vi "target_main.vi"() -> ()   [LabVIEW 2023]
uses:
  <vilib>/Platform/TimedLoop/XDataNode/timing_clust.ctl
  <vilib>/Platform/TimedLoop/XDataNode/nitl_modes.ctl
  <vilib>/Platform/TimedLoop/XDataNode/wakeup.ctl
  <vilib>/rvi/Emulation/niFpgaGetClockAttributes.vi
  <vilib>/rvi/Emulation/niFpgaSctlEmulationGetInTimedLoop.vi
  <vilib>/rvi/Emulation/niFpgaEmulationReportErrorSimple.vi
  <vilib>/rvi/Emulation/niFpgaProcessEmulError.vi
  <vilib>/eio/utilities/niEioResolveVilibRelativePath.vi
  <vilib>/rvi/interface/RandomDataEmulation/niFpgaRandomDataHandleErrors.vi
  <vilib>/rvi/Emulation/niFpgaCriticalErrorInLSC.vi
  <vilib>/rvi/eio/common/nirviEmuTemplateMethod_errors.vi
  <vilib>/rvi/DataTransferAndStorage/Container/XNode/niFpgaContainer.xnode
  <vilib>/rvi/interface/RandomDataEmulation/nirviRandomDataFpgaReadWriteTemplate.vi
  <vilib>/Platform/TimedLoop/XDataNode/XDataNode.xnode
  <vilib>/eio/EIONode/EIONode.xnode
  <vilib>/Platform/TimedLoop/XDataNode/XDNodeRunTimeDep.lvlib
panel:
  out "pin 6":sgl
  out "pin 5":sgl
  out "pin 4":sgl
  out "pin 2":sgl
  out "pin 3":sgl
  out "pin 1":sgl format="%.2f"
  in  "FPGA FIFO Status Update (ms)":u32=100 caption="FPGA FIFO Status Update (mSec)"
  in  "Action Abort":bool
  in  "Status Code":u8
  in  "Analogue 2":u32
  in  "Analogue 1":u32
  in  "Analogue 0":u32
  in  "Digital 0":u32
  in  "Analogue 2 Read":bool
  in  "Analogue 1 Read":bool
  in  "Analogue 0 Read":bool
  in  "Digital 0 Read":bool
  in  "Action: Analogue 2":u64
  in  "Action: Analogue 1":u64
  in  "Action: Analogue 0":u64
  in  "Action: Digital 0":u64
  in  "FPGA Tick Reset":bool
  in  "FPGA Status Update Loop Time (ms)":u32=100 caption="FPGA Execution Status Update (mSec)"
  out "FPGA Target Clock Tick":u32
  # "Current Actions"
  # "Action Execution"
  # "FIFO Read Request"
  # "UDP: FPGA Line Status"
  # "Analogue 0: Optical Switch Pin Status"
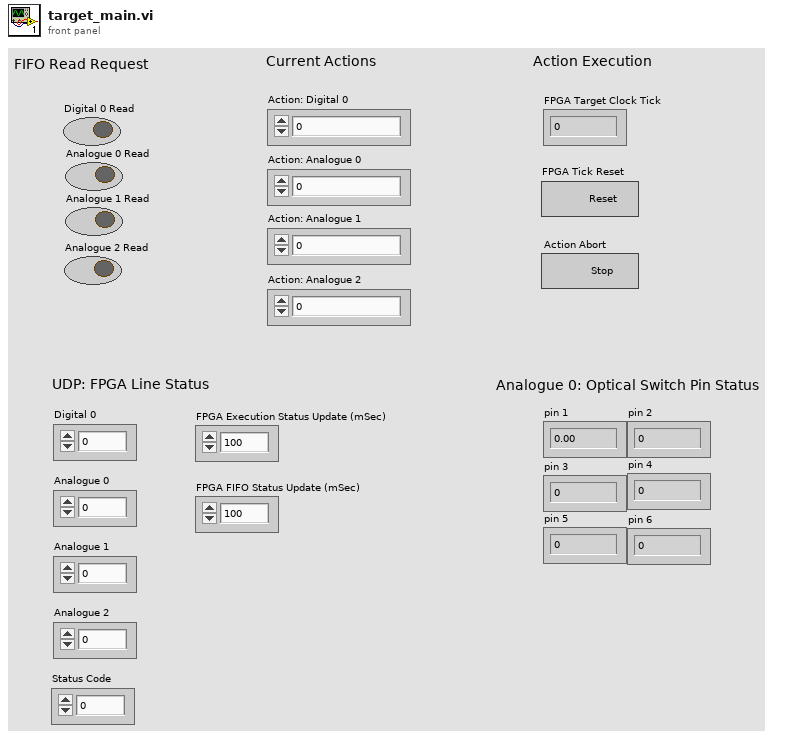
[diagram p1: front panel]
types:
  T1 = typedef "XDNodeRunTimeDep.lvlib/timing_clust.ctl" = cluster{"Expected End [f-1]":u64, "Actual End [f-1]":u64, "Finished Late? [f-1]":bool, "Expected End [i-1]":u64, "Actual End [i-1]":u64, "Finished Late? [i-1]":bool, "Expected Start [i]":u64, "Actual Start [i]":u64, "Expected Start [f]":u64, "Actual Start [f]":u64, "Source Name":string, "Structure Name":string, "Period":i64, "Deadline":i64, "Offset":i64, "Start":i64, "Priority":i32, "Timeout":i32, "Mode":T2, "Wakeup Reason":T3, "Error":errorcluster, "Source Type":string, "Secondary Source Type":string, "Global End Time":u64, "Global Start Time":u64, "Frame Duration":u64, "Iteration Duration":u64, "Assigned CPU":i32, "I/O Scan Engine Mode":u32}
  T2 = typedef "XDNodeRunTimeDep.lvlib/nitl_modes.ctl" = enum32{"No Change", "Process missed periods, maintain original phase", "Discard missed periods, maintain original phase", "Process missed periods, ignore original phase", "Discard missed periods, ignore original phase"}
  T3 = typedef "XDNodeRunTimeDep.lvlib/wakeup.ctl" = enum32{"Normal", "Aborted", "Asynchronous wakeup", "Timing source error", "Timed loop error", "Timeout"}
  T4 = cluster{"pin 1":sgl, "pin 3":sgl, "pin 5":sgl, "pin 6":sgl, "pin 2":sgl, "pin 4":sgl}[]
  T5 = cluster{"pin 1":sgl, "pin 3":sgl, "pin 5":sgl, "pin 6":sgl, "pin 2":sgl, "pin 4":sgl}
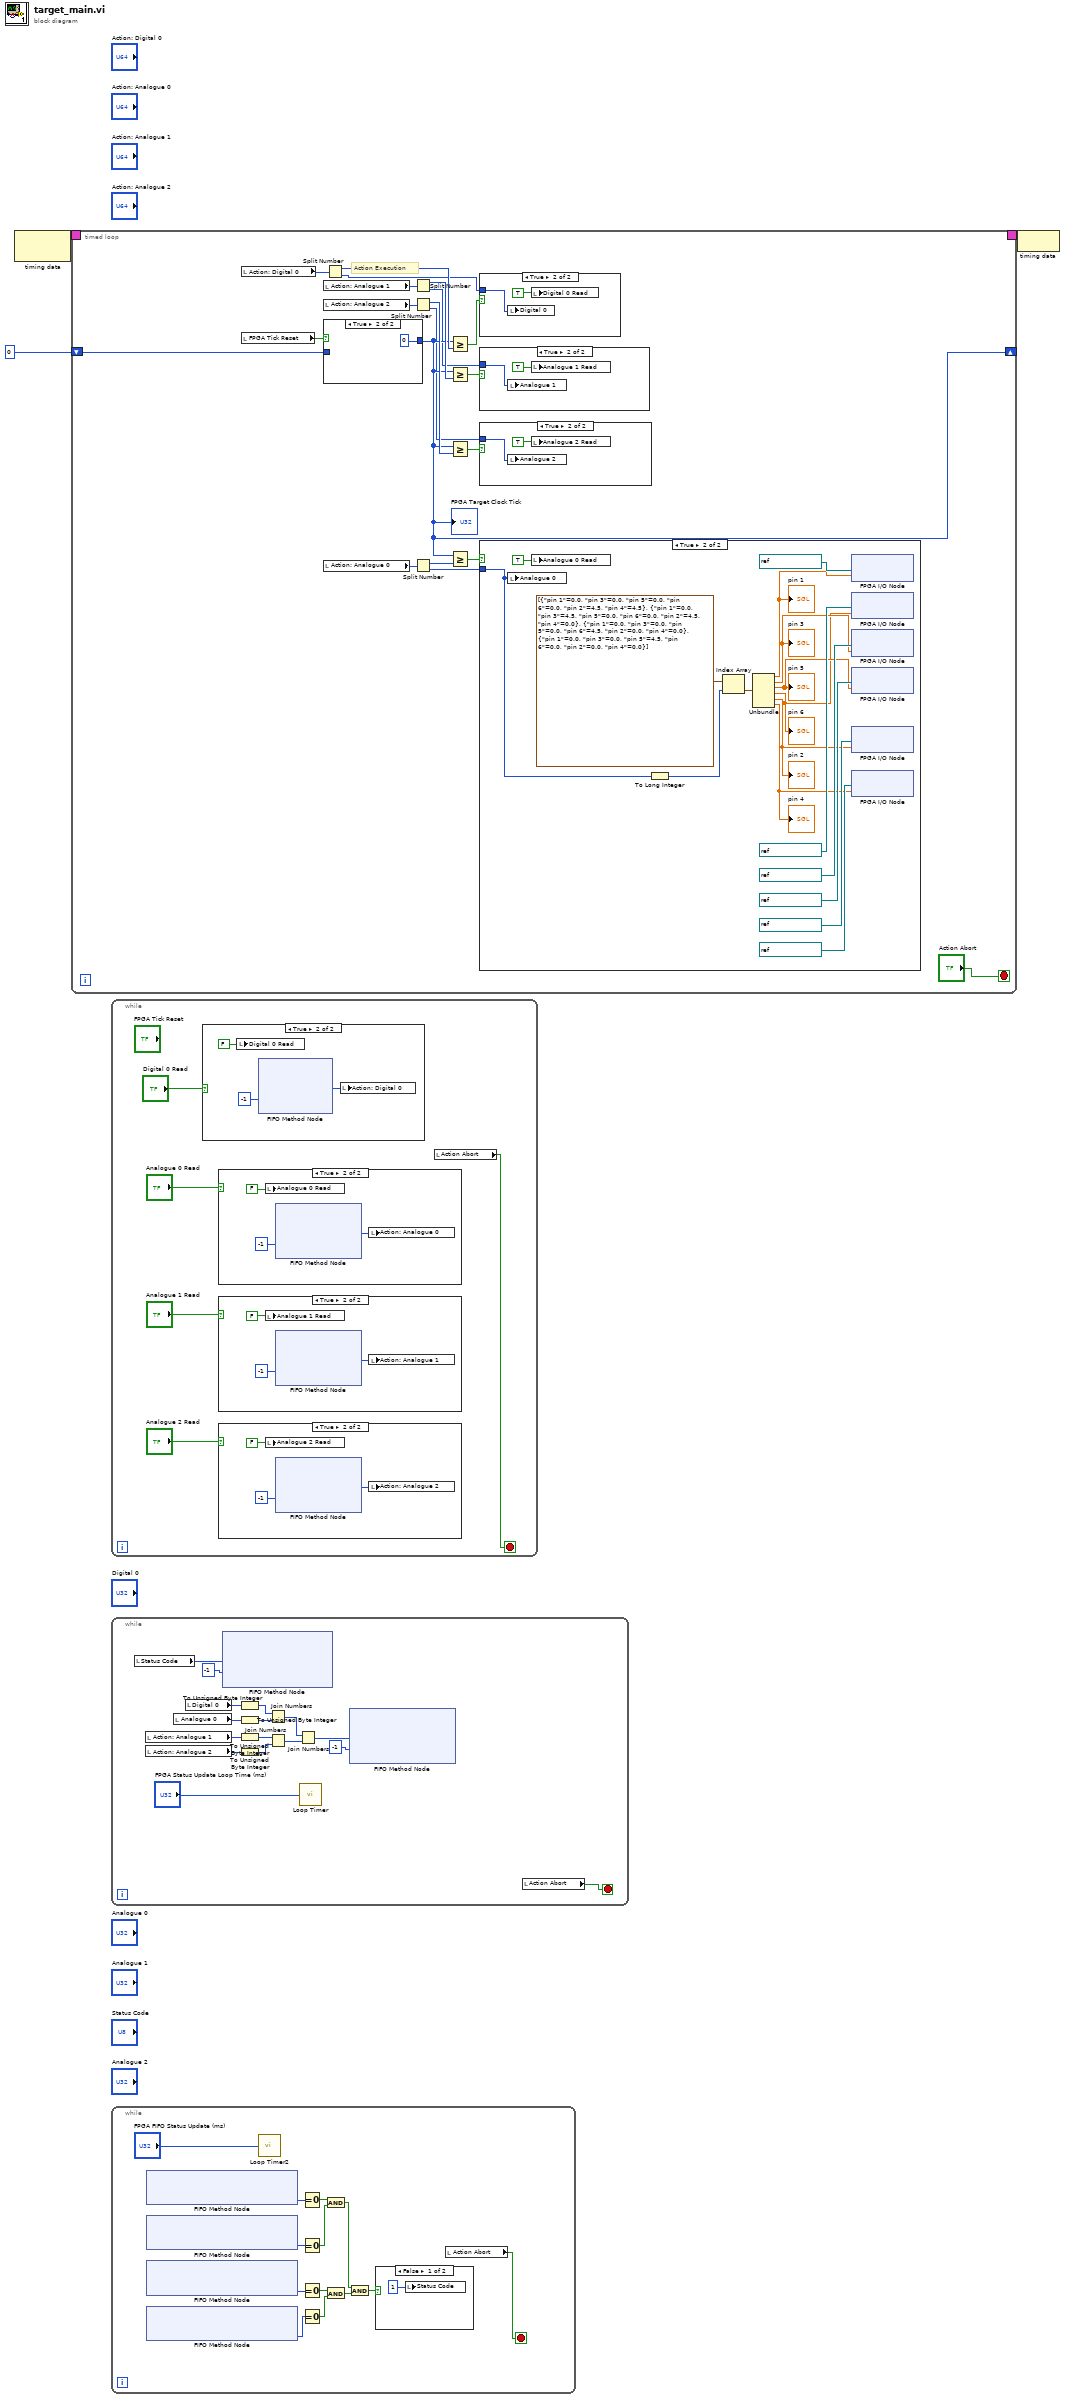
[diagram p0: block diagram]
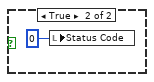
[diagram p2: hidden frame]
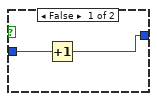
[diagram p7: hidden frame]
diagram:
  n1 = node-c288() -> (w3:T1)  [unwired: 1 in]
  n2 = timed-loop {
    timing: w3 -> [_]
    timing-out: [_] -> w2
    shift-right: [w13] -> _
    shift-left: u32 0 -> [w22]
    stop <- "Action Abort" stop-if-true
    # "Action Execution"
    n3 = local read "Action: Digital 0"() -> (w21:u64)
    n4 = local read "FPGA Tick Reset"() -> (w23:bool)
    n5 = local read "Action: Analogue 1"() -> (w19:u64)
    n6 = local read "Action: Analogue 2"() -> (w18:u64)
    n7 = case shown="True" w23 {
      tunnel: [w48 u32 0] -> w13
      tunnel: w22 -> [w47 _]
      frame False {
        n8 = Increment(x=w47) -> (x+1=w48:u32)
      }
      frame True {
      }
    }
    "FPGA Target Clock Tick" <- w13
    n9 = local read "Action: Analogue 0"() -> (w20:u64)
    n10 = Split Number(x=w21) -> (hi(x)=w17:u32, lo(x)=w11:u32)
    n11 = Split Number(x=w19) -> (hi(x)=w15:u32, lo(x)=w7:u32)
    n12 = Split Number(x=w18) -> (hi(x)=w14:u32, lo(x)=w5:u32)
    n13 = Split Number(x=w20) -> (hi(x)=w16:u32, lo(x)=w9:u32)
    n14 = Greater Or Equal?(x=w13, y=w17) -> (x >= y?=w12:bool)
    n15 = Greater Or Equal?(x=w13, y=w15) -> (x >= y?=w8:bool)
    n16 = Greater Or Equal?(x=w13, y=w14) -> (x >= y?=w6:bool)
    n17 = Greater Or Equal?(x=w13, y=w16) -> (x >= y?=w10:bool)
    n18 = case shown="True" w12 {
      tunnel: w11 -> [_ w46]
      frame False {
      }
      frame True {
        n19 = local write "Digital 0"(w46) -> ()
        n20 = local write "Digital 0 Read"(TRUE) -> ()
      }
    }
    n21 = case shown="True" w8 {
      tunnel: w7 -> [_ w27]
      frame False {
      }
      frame True {
        n22 = local write "Analogue 1"(w27) -> ()
        n23 = local write "Analogue 1 Read"(TRUE ("Analogue 1 Read")) -> ()
      }
    }
    n24 = case shown="True" w6 {
      tunnel: w5 -> [_ w25]
      frame False {
      }
      frame True {
        n25 = local write "Analogue 2"(w25) -> ()
        n26 = local write "Analogue 2 Read"(TRUE ("Analogue 2 Read")) -> ()
      }
    }
    n27 = case shown="True" w10 {
      tunnel: w9 -> [_ w28]
      frame False {
      }
      frame True {
        n28 = local write "Analogue 0"(w28) -> ()
        n29 = local write "Analogue 0 Read"(TRUE ("Analogue 0 Read")) -> ()
        n30 = To Long Integer(number=w28) -> (32bit integer=w29:i32)
        n31 = Index Array(array=T4 [{"pin 1"=0.0, "pin 3"=0.0, "pin 5"=0.0, "pin 6"=0.0, "pin 2"=4.5, "pin 4"=4.5}, {"pin 1"=0.0, "pin 3"=4.5, "pin 5"=0.0, "pin 6"=0.0, "pin 2"=4.5, "pin 4"=0.0}, {"pin 1"=0.0, "pin 3"=0.0, "pin 5"=0.0, "pin 6"=4.5, "pin 2"=0.0, "pin 4"=0.0}, {"pin 1"=0.0, "pin 3"=0.0, "pin 5"=4.5, "pin 6"=0.0, "pin 2"=0.0, "pin 4"=0.0}], index=w29) -> (element=w36:T5)
        n32 = Unbundle(w36) -> ("pin 1"=w35:sgl, "pin 3"=w34:sgl, "pin 5"=w31:sgl, "pin 6"=w30:sgl, "pin 2"=w33:sgl, "pin 4"=w32:sgl)
        "pin 1" <- w35
        "pin 3" <- w34
        "pin 2" <- w33
        "pin 4" <- w32
        "pin 5" <- w31
        "pin 6" <- w30
        n33 = xnode "FPGA I/O Node"("I/O Item"=w35, "FPGA I/O In"=refnum<k21> "Mod3/AO0") -> ()  [unwired: 1 out]
        n34 = xnode "FPGA I/O Node"("I/O Item"=w30, "FPGA I/O In"=refnum<k21> "Mod3/AO5") -> ()  [unwired: 1 out]
        n35 = xnode "FPGA I/O Node"("I/O Item"=w34, "FPGA I/O In"=refnum<k21> "Mod3/AO2") -> ()  [unwired: 1 out]
        n36 = xnode "FPGA I/O Node"("I/O Item"=w31, "FPGA I/O In"=refnum<k21> "Mod3/AO4") -> ()  [unwired: 1 out]
        n37 = xnode "FPGA I/O Node"("I/O Item"=w33, "FPGA I/O In"=refnum<k21> "Mod3/AO1") -> ()  [unwired: 1 out]
        n38 = xnode "FPGA I/O Node"("I/O Item"=w32, "FPGA I/O In"=refnum<k21> "Mod3/AO3") -> ()  [unwired: 1 out]
      }
    }
  }
  n39 = while {
    stop <- w52 stop-if-true
    n40 = case shown="True" "Digital 0 Read" {
      frame False {
      }
      frame True {
        n41 = local write "Digital 0 Read"(FALSE) -> ()
        n42 = xnode ("FIFO Method Node")("Timeout"=-1) -> ("Element"=w68:u64)  [unwired: 1 in, 2 out]
        n43 = local write "Action: Digital 0"(w68) -> ()
      }
    }
    n44 = case shown="True" "Analogue 0 Read" {
      frame False {
      }
      frame True {
        n45 = local write "Analogue 0 Read"(FALSE) -> ()
        n46 = xnode ("FIFO Method Node")("Timeout"=-1) -> ("Element"=w65:u64)  [unwired: 1 in, 2 out]
        n47 = local write "Action: Analogue 0"(w65) -> ()
      }
    }
    n48 = case shown="True" "Analogue 1 Read" {
      frame False {
      }
      frame True {
        n49 = local write "Analogue 1 Read"(FALSE) -> ()
        n50 = xnode ("FIFO Method Node")("Timeout"=-1) -> ("Element"=w62:u64)  [unwired: 1 in, 2 out]
        n51 = local write "Action: Analogue 1"(w62) -> ()
      }
    }
    n52 = case shown="True" "Analogue 2 Read" {
      frame False {
      }
      frame True {
        n53 = local write "Analogue 2 Read"(FALSE) -> ()
        n54 = xnode ("FIFO Method Node")("Timeout"=-1) -> ("Element"=w59:u64)  [unwired: 1 in, 2 out]
        n55 = local write "Action: Analogue 2"(w59) -> ()
      }
    }
    n56 = local read "Action Abort"() -> (w52:bool)
  }
  n57 = while {
    stop <- w81 stop-if-true
    n58 = local read "Status Code"() -> (w82:u8)
    n59 = local read "Action: Analogue 1"() -> (w78:u64)
    n60 = local read "Action: Analogue 2"() -> (w77:u64)
    n61 = local read "Analogue 0"() -> (w79:u32)
    n62 = local read "Digital 0"() -> (w80:u32)
    n63 = xnode ("FIFO Method Node")("Element"=w82, "Timeout"=-1) -> ()  [unwired: 1 in, 2 out]
    n64 = To Unsigned Byte Integer(number=w80) -> (unsigned 8bit integer=w76:u8)
    n65 = To Unsigned Byte Integer(number=w79) -> (unsigned 8bit integer=w75:u8)
    n66 = To Unsigned Byte Integer(number=w78) -> (unsigned 8bit integer=w74:u8)
    n67 = To Unsigned Byte Integer(number=w77) -> (unsigned 8bit integer=w73:u8)
    n68 = Join Numbers(hi=w76, lo=w75) -> ((hi.lo)=w71:u16)
    n69 = Join Numbers(hi=w74, lo=w73) -> ((hi.lo)=w72:u16)
    n70 = Join Numbers(hi=w71, lo=w72) -> ((hi.lo)=w70:u32)
    n71 = call "Loop Timer"("Count(mSec)"="FPGA Status Update Loop Time (ms)") -> ()  [unwired: 1 out]
    n72 = xnode ("FIFO Method Node")("Element"=w70, "Timeout"=-1) -> ()  [unwired: 1 in, 2 out]
    n73 = local read "Action Abort"() -> (w81:bool)
  }
  n74 = while {
    stop <- w97 stop-if-true
    n75 = xnode ("FIFO Method Node")() -> ("Number of Elements to Read"=w96:u32)  [unwired: 1 in, 1 out]
    n76 = xnode ("FIFO Method Node")() -> ("Number of Elements to Read"=w95:u32)  [unwired: 1 in, 1 out]
    n77 = xnode ("FIFO Method Node")() -> ("Number of Elements to Read"=w94:u32)  [unwired: 1 in, 1 out]
    n78 = xnode ("FIFO Method Node")() -> ("Number of Elements to Read"=w93:u32)  [unwired: 1 in, 1 out]
    n79 = call "Loop Timer2"("Count(mSec)"="FPGA FIFO Status Update (ms)") -> ()  [unwired: 1 out]
    n80 = Equal To 0?(x=w96) -> (x = 0?=w92:bool)
    n81 = Equal To 0?(x=w95) -> (x = 0?=w91:bool)
    n82 = Equal To 0?(x=w94) -> (x = 0?=w90:bool)
    n83 = Equal To 0?(x=w93) -> (x = 0?=w89:bool)
    n84 = And(x=w92, y=w91) -> (x .and. y?=w88:bool)
    n85 = And(x=w90, y=w89) -> (x .and. y?=w87:bool)
    n86 = And(x=w88, y=w87) -> (x .and. y?=w86:bool)
    n87 = case shown="False" w86 {
      frame False {
        n88 = local write "Status Code"(u8 1) -> ()
      }
      frame True {
        n89 = local write "Status Code"(u8 0) -> ()
      }
    }
    n90 = local read "Action Abort"() -> (w97:bool)
  }
  n91 = node-c288(w2) -> ()
